vi "SetAnalogOut.vi"(8 "Error in":errorcluster, 9 "Value":dbl, 10 "Signal":refnum<k24>, 11 "DevicesAndSignals":T1) -> (0 "Error out":errorcluster, 3 "DevicesAndSignals":T1)   [LabVIEW 2016]
doc: "Sets the analog out signal to the given value.\n\nSignal: Signal (has to be of type AnalogOutSignal) to adjust\nValue: Value to set"
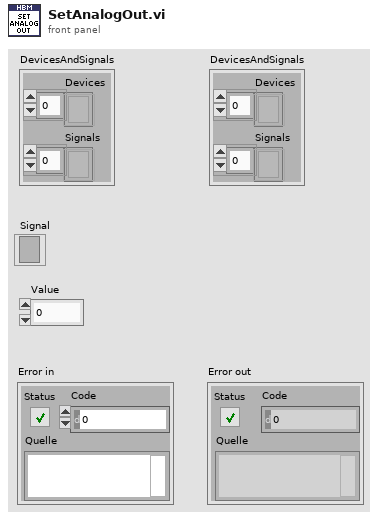
[diagram p1: front panel]
types:
  T1 = cluster{"Devices":refnum<k24>[], "Signals":refnum<k24>[]}
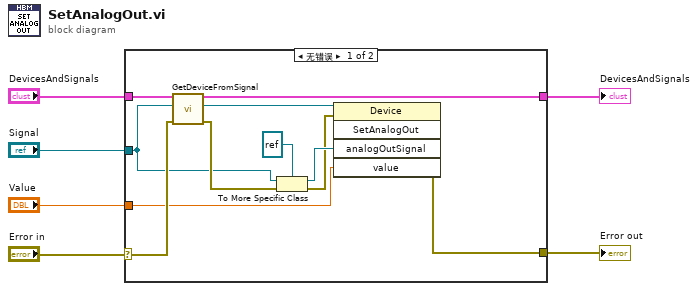
[diagram p0: block diagram]
diagram:
  n1 = case shown="无错误" "Error in" {
    selector: "Error in" -> [w15 w18]
    tunnel: "DevicesAndSignals" -> [w16 w17]
    tunnel: [w8 w18] -> w4
    tunnel: [w7 w17] -> _
    tunnel: "Signal" -> [w9 _]
    tunnel: "Value" -> [w6 _]
    frame No Error {
      n2 = call "GetDeviceFromSignal.vi"("Error in"=w15, "Signal"=w9, "DevicesAndSignals"=w16) -> ("Error out"=w11:errorcluster, "Device"=w14:refnum<k24>, "DevicesAndSignals"=w7:T1)  [unwired: 6 in]
      n3 = To More Specific Class(target class=refnum<k24> refnum ("digitalSignal"), reference=w9, error in=w11) -> (specific class reference=w12:refnum<k24>, error out=w10:errorcluster)
      n4 = invoke on="Methodenknoten" class="Device" method="SetAnalogOut"(reference=w14, error in=w10, "analogOutSignal"=w12, "value"=w6) -> (error out=w8:errorcluster)  [unwired: 1 in, 4 out]
    }
    frame Error {
    }
  }
  "Error out" <- w4
  "DevicesAndSignals" <- "DevicesAndSignals"
